vi "Pivot Module.vi"(0 "pivot":enum16{"FL", "FR", "BL", "BR"}(ring)) -> ()   [LabVIEW 2014]
uses:
  <vilib>/Rock Robotics/WPI/SafetyOutput/WPI_SafetyOutputConfigMenu.ctl
  Begin/Global RefNums.vi
  Begin/Global Variables.vi
  Begin/Global Constants.vi
panel:
  out "s? t:f":dbl
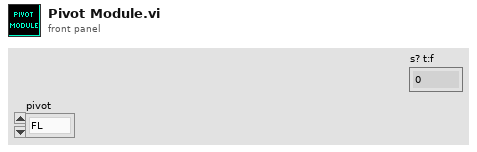
[diagram p1: front panel]
types:
  T1 = typedef "WPI_SafetyOutputConfigMenu.ctl" = enum16{"Enable", "Disable"}
  T2 = typedef "WPI_AnalogChannelDevRef.ctl" = cluster{"DevStatus":errorcluster, "Controller":T3, "Analog Channel":T4}
  T3 = typedef "FPGA_TypedefAnalogModule.ctl" = enum16{"Controller 1"}
  T4 = typedef "FPGA_AIChannel.ctl" = enum8{"AI 0", "AI 1", "AI 2", "AI 3", "AI MXP 0", "AI MXP 1", "AI MXP 2", "AI MXP 3", "Invalid"}
  T5 = cluster{"proportional gain (Kc)":dbl, "integral time (Ti, min)":dbl, "derivative time (Td, min)":dbl}
  T6 = typedef "WPI_MotorControlDeviceRef.ctl" = cluster{"DeviceStatus":errorcluster, "Type":T7, "PWM":cluster{"Controller":T8, "PWM Channel":T9, "DeadBand":T10}, "CAN":cluster{"Device Number":u8, "Control Mode":T11, "Semaphore":T12, "Max Vout":dbl, "TalonSRX Control Mode":T13}, "Invert":bool, "TransformRef":T14, "InvTransformRef":T14}
  T7 = typedef "WPI_MotorControlType.ctl" = enum16{"PWM", "CAN", "CANTalonSRX"}
  T8 = typedef "FPGA_TypedefDigitalModule.ctl" = enum16{"Controller 1"}
  T9 = typedef "FPGA_DIOPWMChannel.ctl" = enum8{"PWM 0", "PWM 1", "PWM 2", "PWM 3", "PWM 4", "PWM 5", "PWM 6", "PWM 7", "PWM 8", "PWM 9", "PWM MXP 0", "PWM MXP 1", "PWM MXP 2", "PWM MXP 3", "PWM MXP 4", "PWM MXP 5", "PWM MXP 6", "PWM MXP 7", "PWM MXP 8", "PWM MXP 9", "Invalid"}
  T10 = typedef "WPI_PWMDeadband.ctl" = cluster{"Name":string, "maxPositivePwm":i32, "minPositivePwm":i32, "centerPwm":i32, "maxNegativePwm":i32, "minNegativePwm":i32, "angularRange":u16}
  T11 = typedef "WPI_CANJaguar_ControlMode.ctl" = enum8{"Percent VBus", "Current", "Speed", "Position", "Voltage"}
  T12 = typedef "Semaphore RefNum" = refnum<k1>
  T13 = typedef "WPI_CANTalonSRX_APIControlMode.ctl" = enum8{"Percent VBus", "Speed", "Position", "Slave", "Unchanged / Invalid"}
  T14 = typedef "WPI_PWMTransform_ConPane.ctl" = refnum<vi>
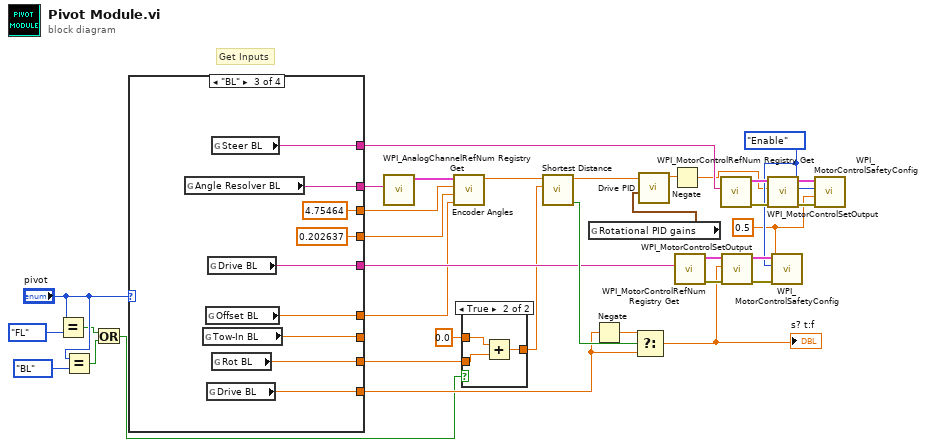
[diagram p0: block diagram]
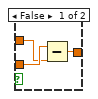
[diagram p2: hidden frame]
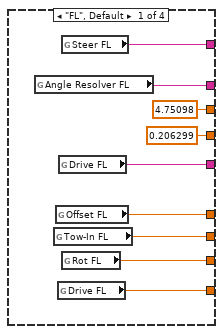
[diagram p3: hidden frame]
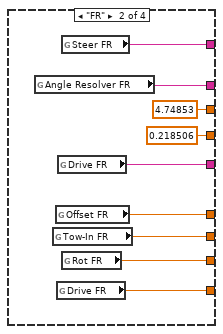
[diagram p4: hidden frame]
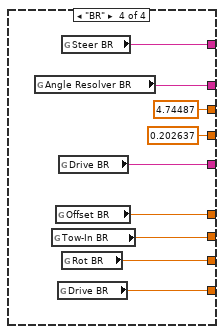
[diagram p5: hidden frame]
diagram:
  w11 = 0.5 ("timeout (s)")
  w24 = WPI_SafetyOutputConfigMenu."Enable" ("mode")
  # "Get Inputs"
  n1 = Equal?(x="pivot", y=enum16{"FL", "FR", "BL", "BR"}."FL") -> (x = y?=w4:bool)
  n2 = Equal?(x="pivot", y=enum16{"FL", "FR", "BL", "BR"}."BL") -> (x = y?=w3:bool)
  n3 = Or(x=w4, y=w3) -> (x .or. y?=w2:bool)
  n4 = case shown="\"BL\"" "pivot" {
    tunnel: [w44 w53 w62 w71] -> w21
    tunnel: [w43 w52 w61 w70] -> w20
    tunnel: [w42 w51 w60 w69] -> w19
    tunnel: [w41 w50 w59 w68] -> w18
    tunnel: [w40 w49 w58 w67] -> w10
    tunnel: [w39 w48 w57 w66] -> w17
    tunnel: [4.75098 ("Resolver BL High Voltage") 4.74853 ("Resolver BL High Voltage") 4.75464 ("Resolver BL High Voltage") 4.74487 ("Resolver BL High Voltage")] -> w16
    tunnel: [0.206299 ("Resolver BL Low Voltage") 0.218506 ("Resolver BL Low Voltage") 0.202637 ("Resolver BL Low Voltage") 0.202637 ("Resolver BL Low Voltage")] -> w15
    tunnel: [w36 w45 w54 w63] -> _
    frame "FL", Default {
      n5 = global read "Global RefNums.vi" "Angle Resolver FL"() -> (w43:string)
      n6 = global read "Global Constants.vi" "Tow-In FL"() -> (w36:dbl)
      n7 = global read "Global Constants.vi" "Offset FL"() -> (w41:dbl)
      n8 = global read "Global Variables.vi" "Drive FL"() -> (w39:dbl)
      n9 = global read "Global RefNums.vi" "Drive FL"() -> (w42:string)
      n10 = global read "Global RefNums.vi" "Steer FL"() -> (w44:string)
      n11 = global read "Global Variables.vi" "Rot FL"() -> (w40:dbl)
    }
    frame "FR" {
      n12 = global read "Global RefNums.vi" "Angle Resolver FR"() -> (w52:string)
      n13 = global read "Global Constants.vi" "Tow-In FR"() -> (w45:dbl)
      n14 = global read "Global Constants.vi" "Offset FR"() -> (w50:dbl)
      n15 = global read "Global Variables.vi" "Drive FR"() -> (w48:dbl)
      n16 = global read "Global RefNums.vi" "Drive FR"() -> (w51:string)
      n17 = global read "Global RefNums.vi" "Steer FR"() -> (w53:string)
      n18 = global read "Global Variables.vi" "Rot FR"() -> (w49:dbl)
    }
    frame "BL" {
      n19 = global read "Global RefNums.vi" "Angle Resolver BL"() -> (w61:string)
      n20 = global read "Global Constants.vi" "Tow-In BL"() -> (w54:dbl)
      n21 = global read "Global Constants.vi" "Offset BL"() -> (w59:dbl)
      n22 = global read "Global Variables.vi" "Drive BL"() -> (w57:dbl)
      n23 = global read "Global RefNums.vi" "Drive BL"() -> (w60:string)
      n24 = global read "Global RefNums.vi" "Steer BL"() -> (w62:string)
      n25 = global read "Global Variables.vi" "Rot BL"() -> (w58:dbl)
    }
    frame "BR" {
      n26 = global read "Global RefNums.vi" "Angle Resolver BR"() -> (w70:string)
      n27 = global read "Global Constants.vi" "Tow-In BR"() -> (w63:dbl)
      n28 = global read "Global Constants.vi" "Offset BR"() -> (w68:dbl)
      n29 = global read "Global Variables.vi" "Drive BR"() -> (w66:dbl)
      n30 = global read "Global RefNums.vi" "Drive BR"() -> (w69:string)
      n31 = global read "Global RefNums.vi" "Steer BR"() -> (w71:string)
      n32 = global read "Global Variables.vi" "Rot BR"() -> (w67:dbl)
    }
  }
  n33 = call <vilib>:"WPI_AnalogChannelRefNum Registry Get.vi"("refnum name"=w20) -> ("AIDeviceRef"=w35:T2)  [unwired: 9 in, 1 out]
  n34 = call "Encoder Angles.vi"("calibration angle"=w18, "low voltage"=w15, "top voltage"=w16, "AIDeviceRef Encoder"=w35) -> ("encoder angle"=w34:dbl)  [unwired: 7 in]
  n35 = case shown="True" w2 {
    tunnel: w10 -> [w73 w77]
    tunnel: 0.0 ("Tow-In BR") -> [w72 w76]
    tunnel: [w74 w75] -> w9
    frame False {
      n36 = Subtract(x=w73, y=w72) -> (x-y=w74:dbl)
    }
    frame True {
      n37 = Add(x=w76, y=w77) -> (x+y=w75:dbl)
    }
  }
  n38 = call "Shortest Distance.vi"("target"=w9, "current"=w34) -> ("flipping?"=w22:bool, "angle to rotate"=w33:dbl)  [unwired: 8 in]
  n39 = global read "Global Constants.vi" "Rotational PID gains"() -> (w12:T5)
  n40 = Negate(x=w17) -> (-x=w23:dbl)
  n41 = Select(t=w23, s=w22, f=w17) -> (s? t:f=w8:dbl)
  "s? t:f" <- w8
  n42 = call "Drive PID.vi"("PID gains"=w12, "Process Variable"=w33) -> ("Output"=w14:dbl)  [unwired: 9 in]
  n43 = Negate(x=w14) -> (-x=w13:dbl)
  n44 = call <vilib>:"WPI_MotorControlRefNum Registry Get.vi"("refnum name"=w19) -> ("error out"=w28:errorcluster, "MotorControlDevRef"=w27:T6)  [unwired: 9 in]
  n45 = call <vilib>:"WPI_MotorControlRefNum Registry Get.vi"("refnum name"=w21) -> ("error out"=w32:errorcluster, "MotorControlDevRef"=w31:T6)  [unwired: 9 in]
  n46 = call <vilib>:"WPI_MotorControlSetOutput.vi"("error in (no error)"=w28, "Output"=w8, "MotorControlDevRef"=w27) -> ("error out"=w26:errorcluster, "MotorControlDevRef"=w25:T6)  [unwired: 6 in, 1 out]
  n47 = call <vilib>:"WPI_MotorControlSetOutput.vi"("error in (no error)"=w32, "Output"=w13, "MotorControlDevRef"=w31) -> ("error out"=w30:errorcluster, "MotorControlDevRef"=w29:T6)  [unwired: 6 in, 1 out]
  n48 = call <vilib>:"WPI_MotorControlSafetyConfig.vi"("error in (no error)"=w26, "timeout (s)"=w11, "mode"=w24, "MotorControlDevRef"=w25) -> ()  [unwired: 6 in, 2 out]
  n49 = call <vilib>:"WPI_MotorControlSafetyConfig.vi"("error in (no error)"=w30, "timeout (s)"=w11, "mode"=w24, "MotorControlDevRef"=w29) -> ()  [unwired: 6 in, 2 out]
